vi "beginPrepareKeeperPassPlay.vi"(8 "error in (no error)":errorcluster, 9 "command_interpreted":T1, 10 "Game in":refnum<class "Game.lvclass">, 11 "PrepareKeeperPassPlay in":refnum<class "PrepareKeeperPassPlay.lvclass">) -> (0 "error out":errorcluster, 2 "begin ?":bool, 3 "PrepareKeeperPassPlay out":refnum<class "PrepareKeeperPassPlay.lvclass">)   [LabVIEW 2021, in "PrepareKeeperPassPlay.lvclass"]
uses:
  PrepareKeeperPassPlay.lvclass
  Game_class/Game.lvclass
  Referee_class/command_interpreted.ctl
  Team_class/OffensivePlay.ctl
  Game_class/Game.lvclass/Game.ctl
  Team_class/Team.lvclass/Team.ctl
  Object_class/Object.lvclass/Object.ctl
  Game_class/Read OffensiveTeam.vi
  Game_class/Read BallRef.vi
  Game_class/Read Utilities.lvclass.vi
  Object_class/Read x.vi
  Object_class/Read y.vi
  Team_class/Read OffensivePlay.vi
  Ball_class/Ball.lvclass
  D:/RoboIme/horie/SSL_AI/Object_class/Object.lvclass
  Ally_class/Ally.lvclass
  D:/RoboIme/horie/SSL_AI/Team_class/Team.lvclass
  Utilities_class/Utilities.lvclass
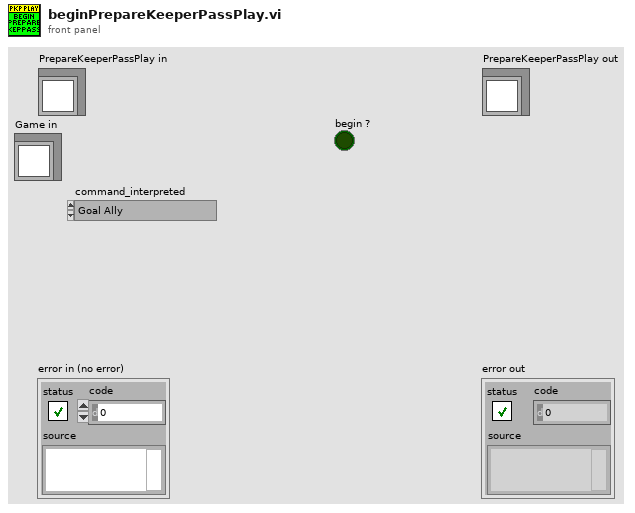
[diagram p1: front panel]
types:
  T1 = typedef "command_interpreted.ctl" = enum16{"Goal Ally", "Goal Enemy", "Ball Placement Enemy", "Ball Placement Ally", "Normal Half Time", "Extra Time  Break", "Extra Half Time", "None", "Post Game", "PKA Normal Start", "Prepare Kickoff Ally", "PKE Normal Start", "Prepare Kickoff Enemy", "Force Start", "Halt", "Timeout", "Prepare Penalty Ally", "Prepare Penalty Enemy", "PPA NormalStart", "PPE Normal Start", "Indirect Free Ally", "Direct Free Enemy", "Direct Free Ally", "Indirect Free Enemy", "Stop"}
  T2 = typedef "OffensivePlay.ctl" = enum16{"5RobotsPassGamePlay", "5PreparePassGame", "5RobotsKeeperGame", "KeeperPassToStriker", "5RobotsNormalGamePlay", "PrepareKeeperPass", "ACBPass", "ABCPass", "PrepareTriplePass", "TableWithStriker", "TableWith2ndStrikerPlay", "PrepareDoublePass", "PrepareRollToPass", "SimplePass", "PreparePass", "PassToStriker", "BallOutOfField", "PassTo2ndStriker", "StopOffensive", "Prepare Penalty Enemy", "EnemyPossessionAtEnemyField", "EnemyPossesionAtOurField", "TestPlay", "PreparePenaltyAlly", "KickPenaltyAlly", "PrepareKickoffAlly", "PrepareKickoffEnemy", "IndirectEnemy", "DirectEnemy", "PreparePassInGame1", "NormalGame", "DirectKick", "Pass", "Halt", "Timeout", "PassPlay", "PenaltyEnemy"}
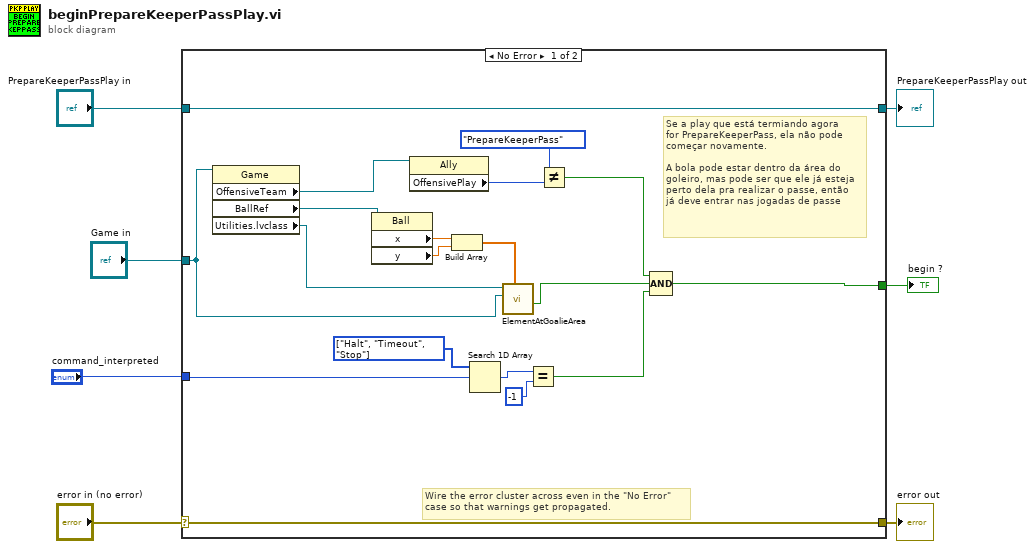
[diagram p0: block diagram]
diagram:
  n1 = case shown="No Error" "error in (no error)" {
    selector: "error in (no error)" -> [w25 w28]
    tunnel: [w25 w28] -> w6
    tunnel: [w26 w27] -> w4
    tunnel: "PrepareKeeperPassPlay in" -> [w26 w27]
    tunnel: "Game in" -> [w24 _]
    tunnel: [w18 _] -> w1
    tunnel: "command_interpreted" -> [w14 _]
    frame No Error {
      w17 = T1[] [enum."Halt", enum."Timeout", enum."Stop"] items=["Goal Ally", "Goal Enemy", "Ball Placement Enemy", "Ball Placement Ally", "Normal Half Time", "Extra Time  Break", "Extra Half Time", "None", "Post Game", "PKA Normal Start", "Prepare Kickoff Ally", "PKE Normal Start", "Prepare Kickoff Enemy", "Force Start", "Halt", "Timeout", "Prepare Penalty Ally", "Prepare Penalty Enemy", "PPA NormalStart", "PPE Normal Start", "Indirect Free Ally", "Direct Free Enemy", "Direct Free Ally", "Indirect Free Enemy", "Stop"] ("Array")
      # "Se a play que está termiando agora\nfor PrepareKeeperPass, ela não pode\ncomeçar novamente.\n\nA bola pode estar dentro da área do\ngoleiro, mas pode ser que ele já esteja\nperto dela pra realizar o passe, então\njá deve entrar nas jogadas de passe"
      # "Wire the error cluster across even in the \"No Error\"\ncase so that warnings get propagated."
      n2 = property class="Game"(reference=w24) -> ("OffensiveTeam"=w9:refnum<class "Ally.lvclass">, "BallRef"=w23:refnum<class "Ball.lvclass">, "Utilities.lvclass"=w8:refnum<class "Utilities.lvclass">)  [unwired: 1 in, 2 out]
      n3 = property class="Ball"(reference=w23) -> ("x"=w22:dbl, "y"=w21:dbl)  [unwired: 1 in, 2 out]
      n4 = property class="Ally"(reference=w9) -> ("OffensivePlay"=w12:T2)  [unwired: 1 in, 2 out]
      n5 = Build Array(w22, w21) -> (w20:dbl[])
      n6 = Search 1D Array(1D array=w17, element=w14) -> (index of element=w16:i32)  [unwired: 1 in]
      n7 = call "ElementAtGoalieArea.vi"("Elemento pos."=w20, "Game"=w24, "Utilities in"=w8) -> ("Element at our goalkeeper area ?"=w19:bool)  [unwired: 4 in, 4 out]
      n8 = Equal?(x=w16, y=-1) -> (x = y?=w13:bool)
      n9 = Not Equal?(x=OffensivePlay."PrepareKeeperPass", y=w12) -> (x != y?=w10:bool)
      n10 = Compound Arithmetic op=AND(w10, w19, w13) -> (w18:bool)
    }
    frame Error {
    }
  }
  "error out" <- w6
  "PrepareKeeperPassPlay out" <- w4
  "begin ?" <- w1
